vi "Write Identifier.vi"(0 "Session Handle In":T1, 5 "identifier":u16, 11 "error in (no error)":errorcluster) -> (4 "Session Handle Out":T1, 15 "error out":errorcluster)   [LabVIEW 2015, in "Peltier.lvclass"]
uses:
  Peltier.lvclass
  Typedefs/Session Handle.ctl
  Peltier.lvclass/Peltier.ctl
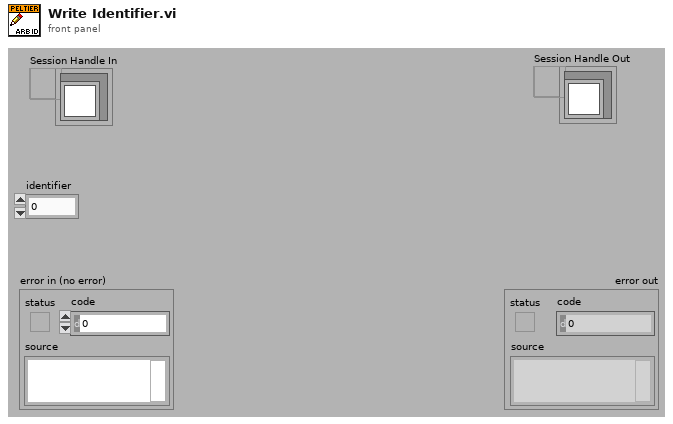
[diagram p1: front panel]
types:
  T1 = typedef "Peltier.lvclass/Session Handle.ctl" = refnum<data-value>
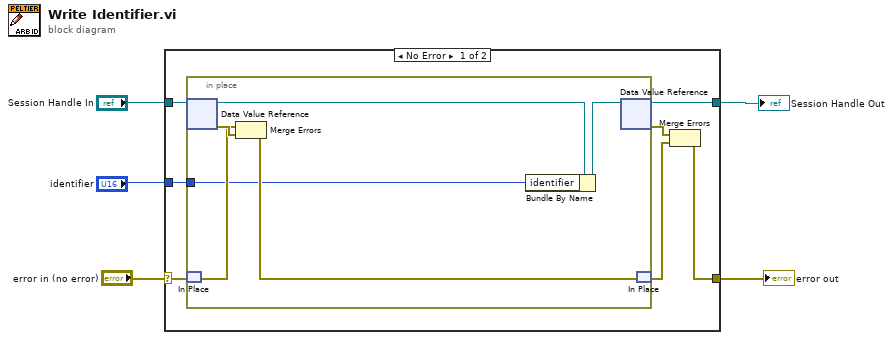
[diagram p0: block diagram]
diagram:
  n1 = case shown="No Error" "error in (no error)" {
    selector: "error in (no error)" -> [w7 w19]
    tunnel: "Session Handle In" -> [w12 w20]
    tunnel: [w11 w20] -> w2
    tunnel: [w8 w19] -> w5
    tunnel: "identifier" -> [w6 _]
    frame No Error {
      n2 = in-place {
        in-place-border: w6 -> [w15]
        n3 = in-place-dvr #1(w12) -> (w14:refnum<class "Peltier.lvclass">, w17:errorcluster)
        n4 = in-place-match #2(w7) -> (w16:errorcluster)
        n5 = Merge Errors(w16, w17) -> (w18:errorcluster)
        n6 = Bundle By Name(cluster=w14, "identifier"=w15) -> (w13:refnum<class "Peltier.lvclass">)
        n7 = in-place-dvr #1(w13) -> (w11:T1, w9:errorcluster)
        n8 = in-place-match #2(w18) -> (w10:errorcluster)
      }
      n9 = Merge Errors(w9, w10) -> (w8:errorcluster)
    }
    frame Error {
    }
  }
  "error out" <- w5
  "Session Handle Out" <- w2
